vi "Color control.vi"() -> ()   [LabVIEW 2017]
panel:
  in  "Stop Button":bool
  in  "Change color":u16(ring) items=["Bleu", "Blanc", "Rouge"]
  in  "Slide":dbl(slide) scale=0.0..10.0
  # "Para cambiar el color del fondo:\n\nshift+click derecho, abre barra de herramientas. luego clic derecho para seleccionar el color.\n\ny shift + click derecho y selecconar las herramientas para volver al estado normal."
  # "Desactivar cuadricula: tools> options> Front Panel, Desactivar opcion Show front panel grid"
  # "Para cambiar color del Controlador del Slider Create>Property Node > Slider colors > FG color\ny se le cambia el tamaño en Advanced > Customize"
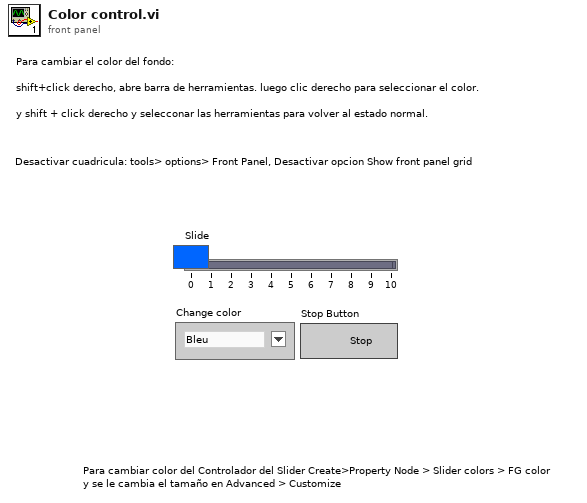
[diagram p1: front panel]
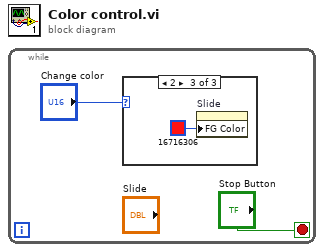
[diagram p0: block diagram]
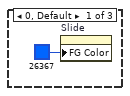
[diagram p2: hidden frame]
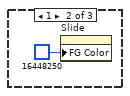
[diagram p3: hidden frame]
diagram:
  n1 = while {
    stop <- "Stop Button" stop-if-true
    n2 = case shown="2" "Change color" {
      frame 0, Default {
        n3 = property on="Slide" class="Slide (strict)"("FG Color"=u32 26367 ("Color Box")) -> ()  [unwired: 2 in, 2 out]
      }
      frame 1 {
        n4 = property on="Slide" class="Slide (strict)"("FG Color"=u32 16448250 ("Color Box")) -> ()  [unwired: 2 in, 2 out]
      }
      frame 2 {
        n5 = property on="Slide" class="Slide (strict)"("FG Color"=u32 16716306 ("Color Box")) -> ()  [unwired: 2 in, 2 out]
      }
    }
  }
